vi "Terminal-DAQ-6133-Getter.vi"(8 "error in (no error)":errorcluster caption="错误输入（无错误）", 10 "读取次数":i32=160, 11 "write operation timeout (ms)":i32=5000 caption="写操作超时（5000毫秒）") -> (0 "error out":errorcluster caption="错误输出", 3 "6133":T1)   [LabVIEW 2014]
panel:
  in  "最大失败次数":i32=5
  out "失败次数":i32
  out "读取次数 2":i32
  in  "最大失败次数":i32=5
  in  "读取次数":i32=161
  out "error out":errorcluster caption="错误输出"
  in  "error in (no error)":errorcluster caption="错误输入（无错误）"
  in  "write operation timeout (ms)":i32=5000 caption="写操作超时（5000毫秒）"
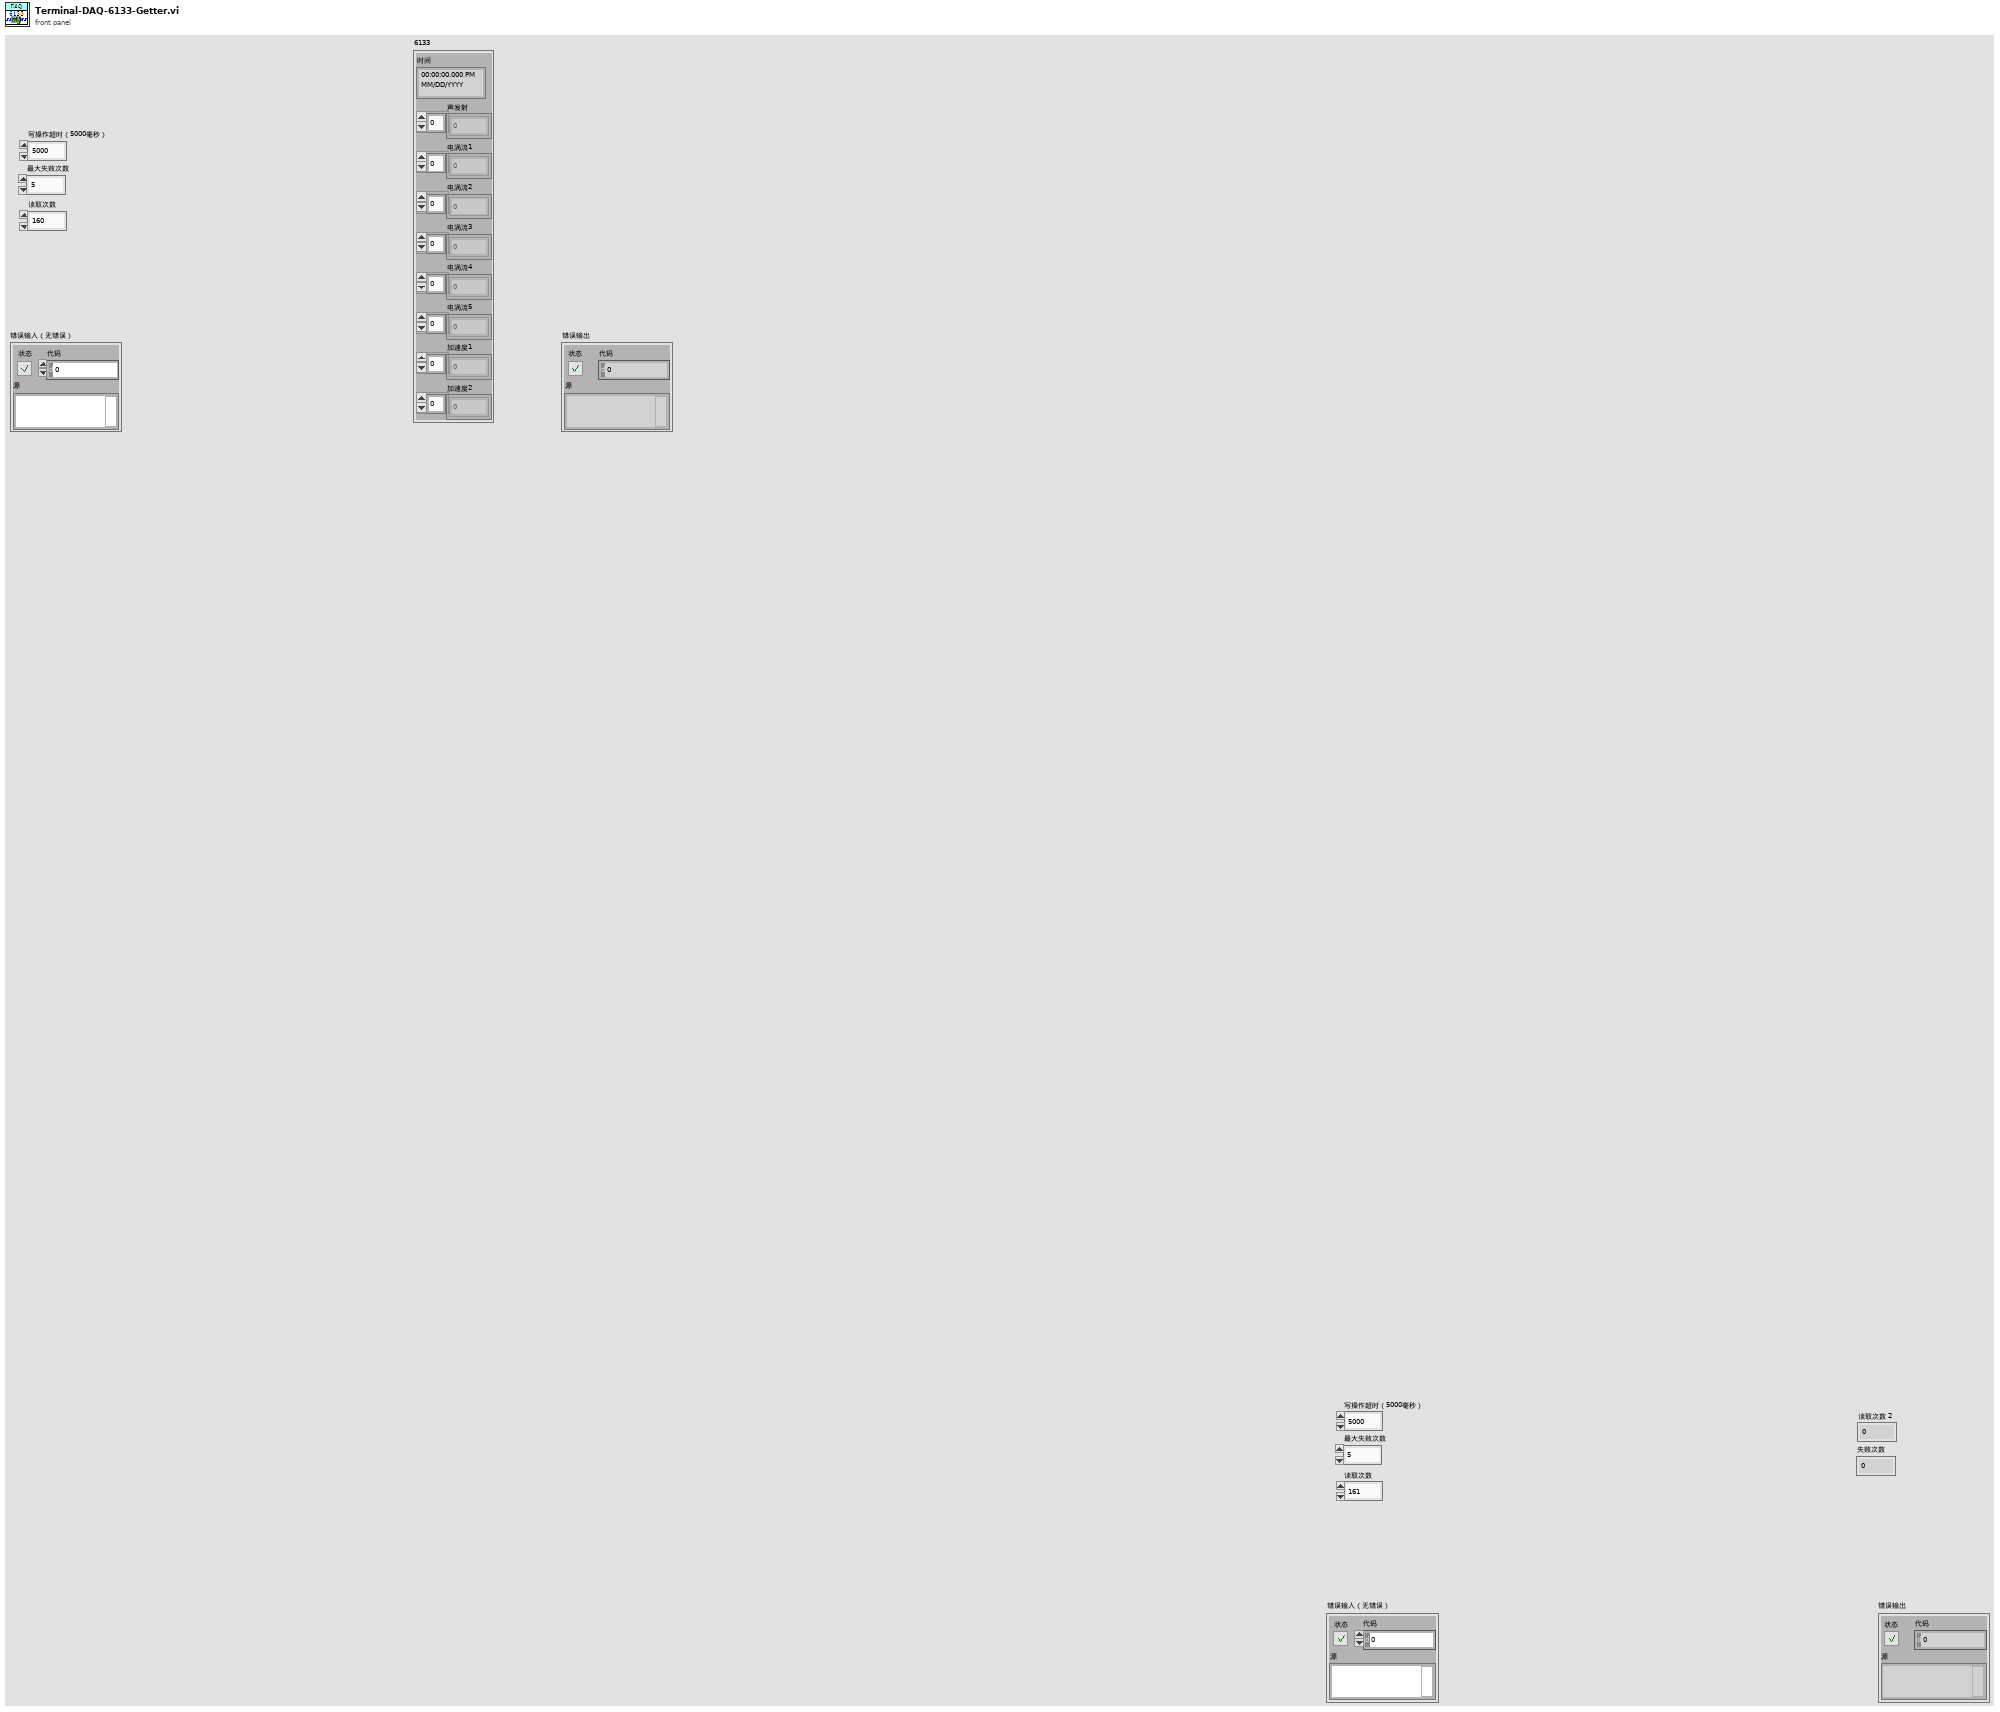
[diagram p1: front panel]
types:
  T1 = cluster{"时间":timestamp, "声发射":sgl[], "电涡流1":sgl[], "电涡流2":sgl[], "电涡流3":sgl[], "电涡流4":sgl[], "电涡流5":sgl[], "加速度1":sgl[], "加速度2":sgl[]}
  T2 = cluster{"设备名":string, "时间":timestamp, "数据":sgl[][], "通道长度":i32[], "次数":i32}
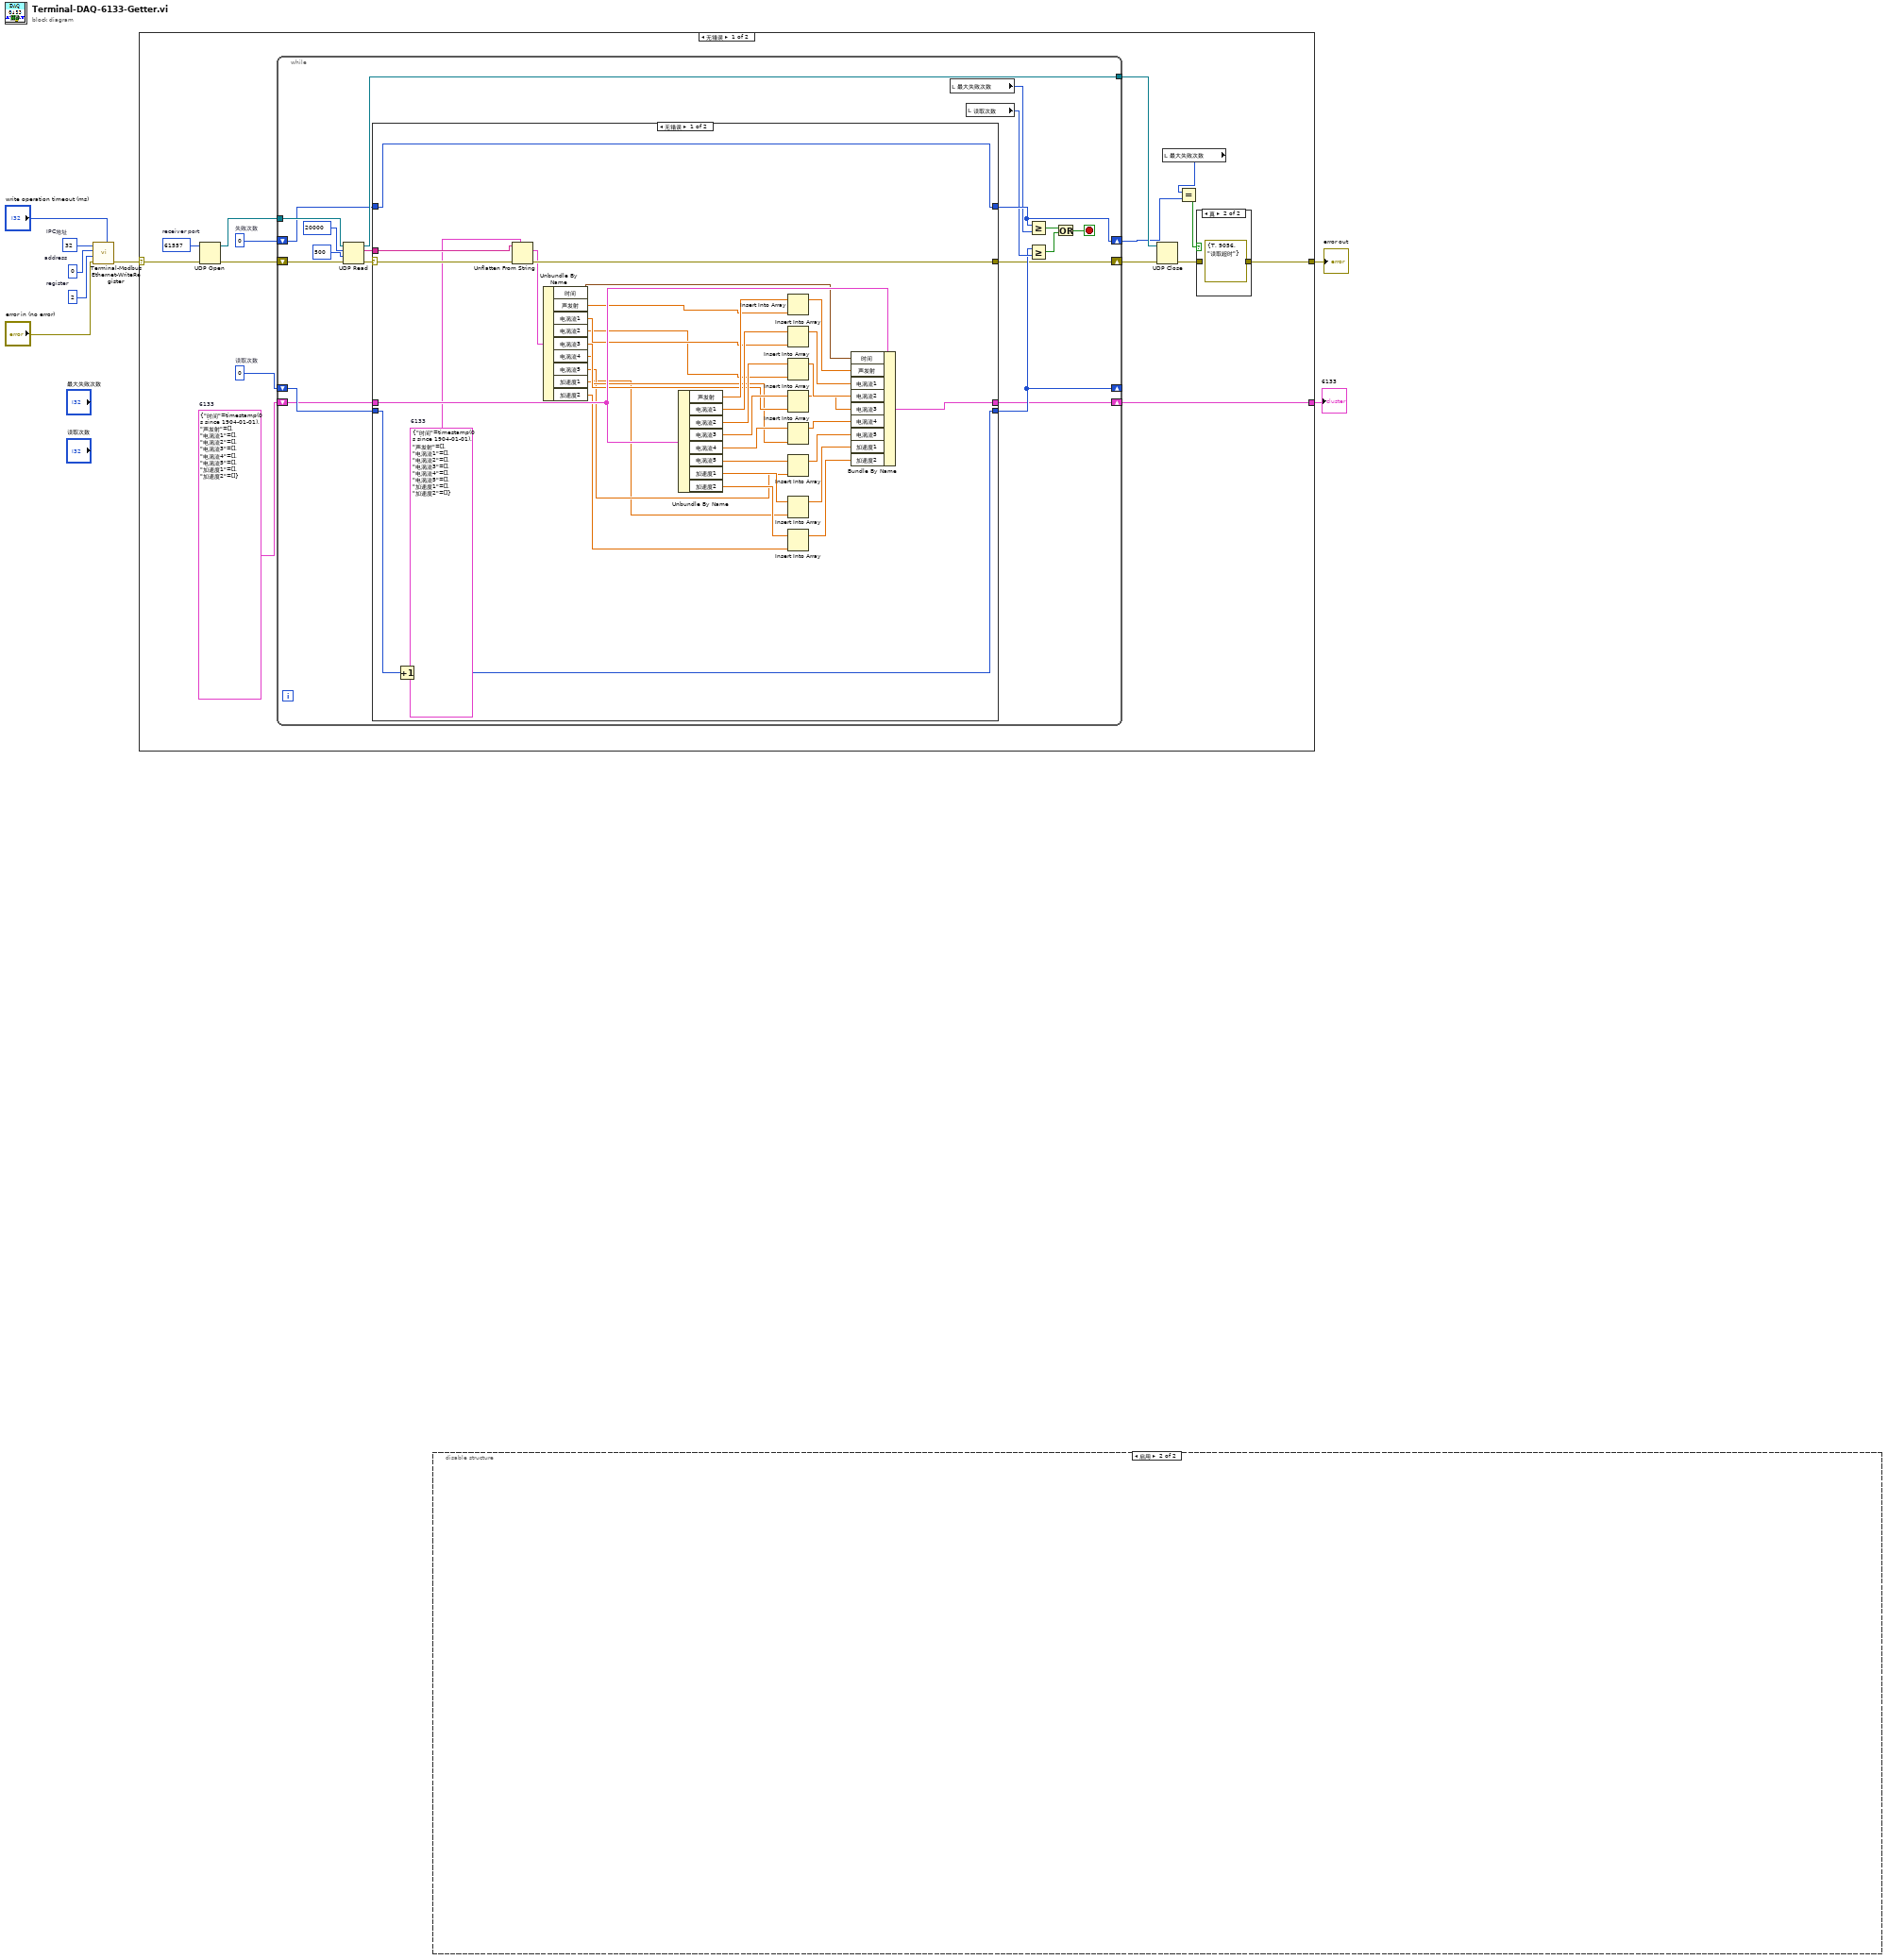
[diagram p0: block diagram]
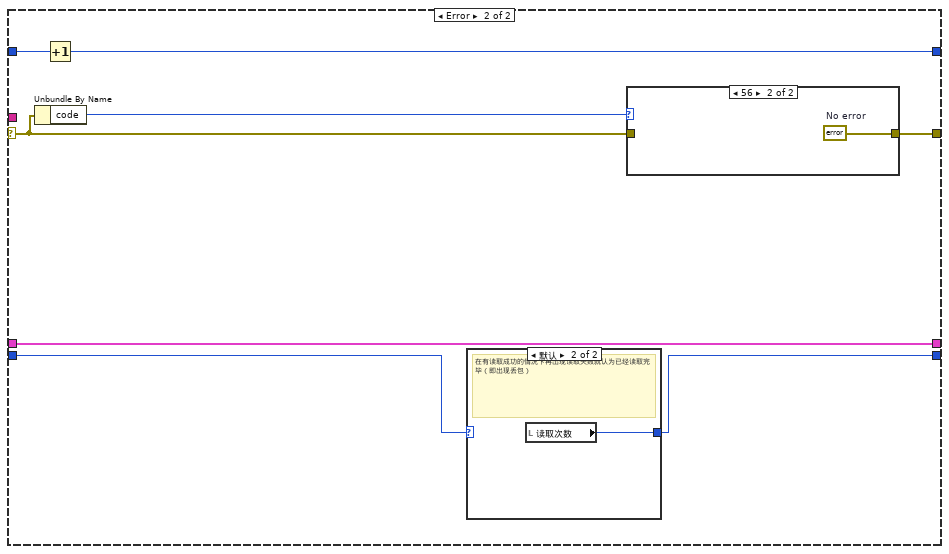
[diagram p3: hidden frame]
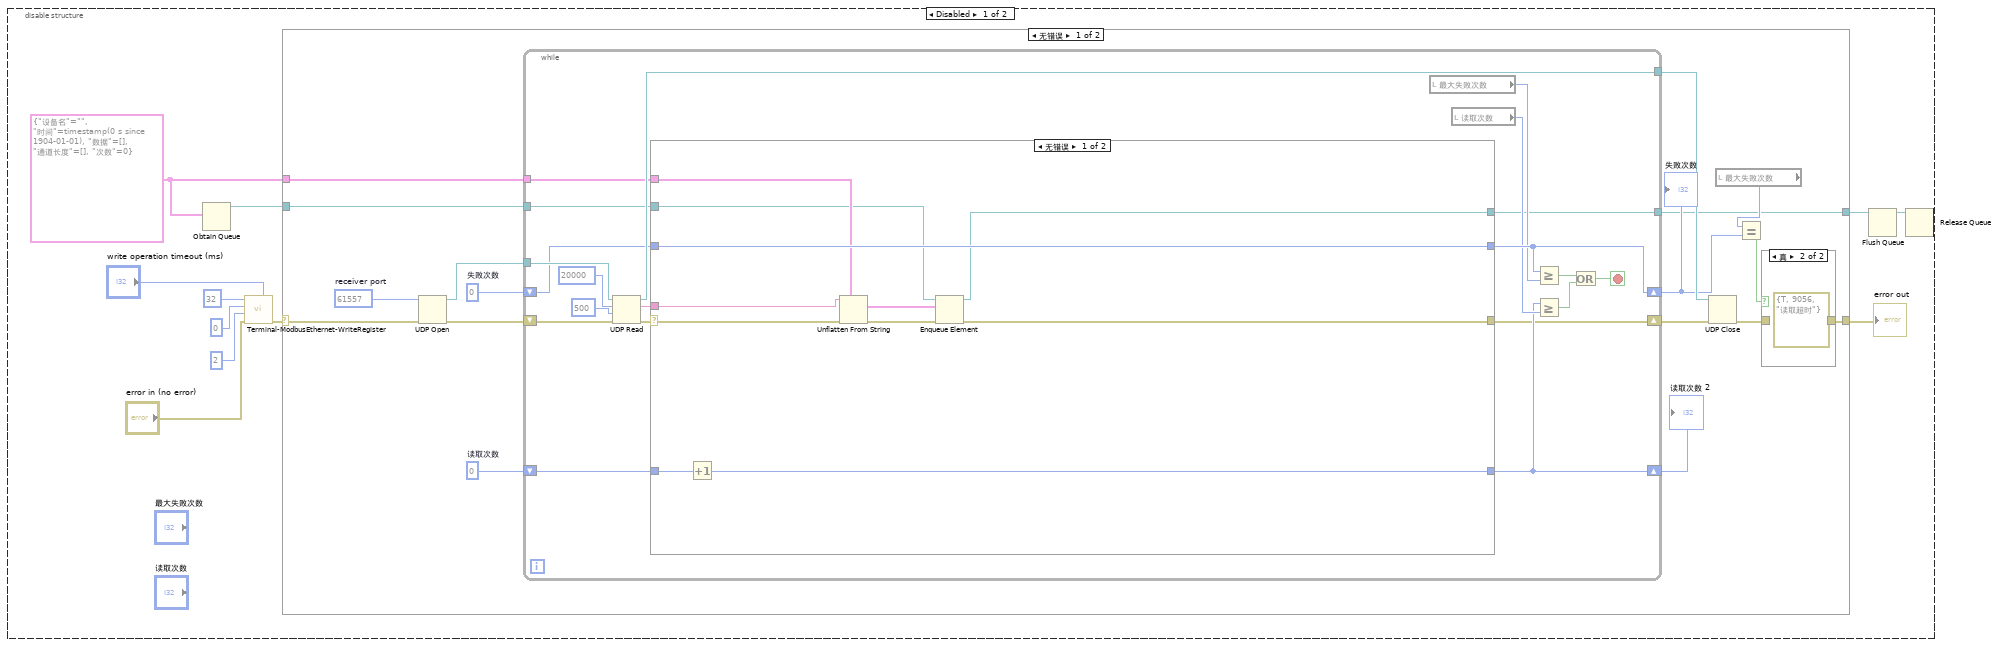
[diagram p7: hidden frame]
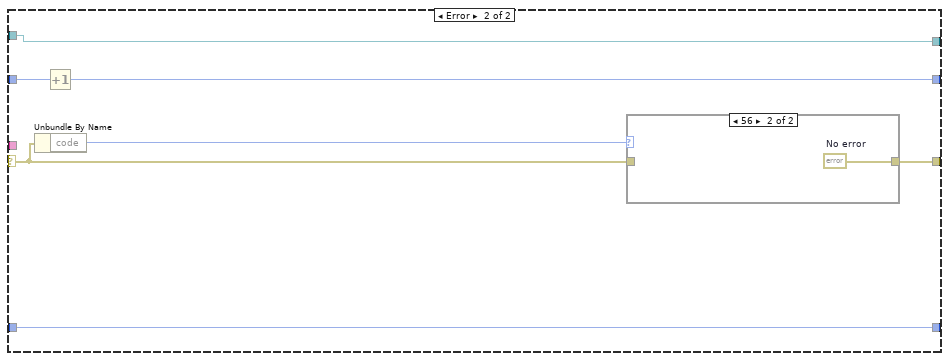
[diagram p9: hidden frame]
diagram:
  w4 = u16 2  # register
  w6 = u16 0  # address
  w5 = u8 32  # IPC地址
  n1 = call "Terminal-ModbusEthernet-WriteRegister.vi"("write operation timeout (ms)"="write operation timeout (ms)", "error in"="error in (no error)", "holding register value"=w4, "address"=w6, "unit ID"=w5) -> ("error out"=w3:errorcluster)  [unwired: 6 in]
  n2 = case shown="无错误" w3 {
    selector: w3 -> [w16 w92]
    tunnel: [w11 w92] -> w2
    tunnel: [w9 _] -> w1
    frame No Error {
      w10 = T1 {"时间"=timestamp(0 s since 1904-01-01), "声发射"=[], "电涡流1"=[], "电涡流2"=[], "电涡流3"=[], "电涡流4"=[], "电涡流5"=[], "加速度1"=[], "加速度2"=[]}  # 6133
      w17 = 0  # 读取次数
      w18 = 0  # 失败次数
      w23 = u16 61557  # receiver port
      n3 = UDP Open(8:w16, 11:w23) -> (port=w22:refnum<k16>, 0:w21:errorcluster)  [unwired: 3 in, 1 out]
      n4 = while {
        tunnel: w22 -> [w42]
        shift-right: [w28] -> w20
        shift-left: w21 -> [w41]
        tunnel: [w39] -> w19
        shift-right: [w36] -> w14
        shift-left: w18 -> [w37]
        shift-right: [w29] -> _
        shift-left: w17 -> [w35]
        shift-right: [w26] -> w9
        shift-left: w10 -> [w27]
        stop <- w31 stop-if-true
        n5 = UDP Read(connection ID=w42, max size (548)=20000 ("最大值(548)"), timeout ms (25000)=500, 8:w41) -> (data out=w38:string, error out=w40:errorcluster, 3:w39:refnum<k16>)  [unwired: 2 out]
        n6 = case shown="无错误" w40 {
          selector: w40 -> [w75 w85]
          tunnel: w38 -> [w79 _]
          tunnel: [w74 w86] -> w28
          tunnel: w37 -> [w76 w84]
          tunnel: [w76 w83] -> w36
          tunnel: w35 -> [w78 w81]
          tunnel: [w77 w80] -> w29
          tunnel: w27 -> [w73 w82]
          tunnel: [w71 w82] -> w26
          frame No Error {
            w53 = T1 {"时间"=timestamp(0 s since 1904-01-01), "声发射"=[], "电涡流1"=[], "电涡流2"=[], "电涡流3"=[], "电涡流4"=[], "电涡流5"=[], "加速度1"=[], "加速度2"=[]}  # 6133
            n7 = Increment(x=w78) -> (x+1=w77:i32)
            n8 = Unflatten From String(type=w53, binary string=w79, error in (no error)=w75) -> (value=w72:T1, error out=w74:errorcluster)  [unwired: 2 in, 1 out]
            n9 = Unbundle By Name(w72) -> ("时间"=w54:timestamp, "声发射"=w52:sgl[], "电涡流1"=w51:sgl[], "电涡流2"=w50:sgl[], "电涡流3"=w49:sgl[], "电涡流4"=w48:sgl[], "电涡流5"=w47:sgl[], "加速度1"=w46:sgl[], "加速度2"=w45:sgl[])
            n10 = Unbundle By Name(w73) -> ("声发射"=w70:sgl[], "电涡流1"=w69:sgl[], "电涡流2"=w68:sgl[], "电涡流3"=w67:sgl[], "电涡流4"=w66:sgl[], "电涡流5"=w65:sgl[], "加速度1"=w64:sgl[], "加速度2"=w63:sgl[])
            n11 = Insert Into Array(array=w70, new element=w52) -> (w55:sgl[])  [unwired: 1 in]
            n12 = Insert Into Array(array=w69, new element=w51) -> (w62:sgl[])  [unwired: 1 in]
            n13 = Insert Into Array(array=w68, new element=w50) -> (w61:sgl[])  [unwired: 1 in]
            n14 = Insert Into Array(array=w67, new element=w49) -> (w60:sgl[])  [unwired: 1 in]
            n15 = Insert Into Array(array=w66, new element=w48) -> (w59:sgl[])  [unwired: 1 in]
            n16 = Insert Into Array(array=w65, new element=w47) -> (w58:sgl[])  [unwired: 1 in]
            n17 = Insert Into Array(array=w64, new element=w46) -> (w57:sgl[])  [unwired: 1 in]
            n18 = Insert Into Array(array=w63, new element=w45) -> (w56:sgl[])  [unwired: 1 in]
            n19 = Bundle By Name(cluster=w73, "时间"=w54, "声发射"=w55, "电涡流1"=w62, "电涡流2"=w61, "电涡流3"=w60, "电涡流4"=w59, "电涡流5"=w58, "加速度1"=w57, "加速度2"=w56) -> (w71:T1)
          }
          frame Error {
            n20 = Unbundle By Name(w85) -> ("code"=w87:i32)
            n21 = Increment(x=w84) -> (x+1=w83:i32)
            n22 = case shown="默认" w81 {
              selector: w81 -> [w88 _]
              tunnel: [w88 w89] -> w80
              frame 0 {
              }
              frame Default {
                # "在有读取成功的情况下再出现读取失败就认为已经读取完毕（即出现丢包）"
                n23 = local read "读取次数"() -> (w89:i32)
              }
            }
            n24 = case shown="56" w87 {
              tunnel: w85 -> [w90 _]
              tunnel: [w90 w91] -> w86
              frame Default {
              }
              frame 56 {
                w91 = errorcluster {"status"=FALSE, "code"=0, "source"=""}  # No error
              }
            }
          }
        }
        n25 = local read "最大失败次数"() -> (w30:i32)
        n26 = local read "读取次数"() -> (w34:i32)
        n27 = Greater Or Equal?(x=w36, y=w30) -> (x >= y?=w33:bool)
        n28 = Greater Or Equal?(x=w29, y=w34) -> (x >= y?=w32:bool)
        n29 = Or(x=w33, y=w32) -> (x .or. y?=w31:bool)
      }
      n30 = UDP Close(connection ID=w19, 8:w20) -> (error out=w12:errorcluster)  [unwired: 1 out]
      n31 = local read "最大失败次数"() -> (w15:i32)
      n32 = Equal?(x=w15, y=w14) -> (x = y?=w13:bool)
      n33 = case shown="真" w13 {
        tunnel: w12 -> [w24 _]
        tunnel: [w24 errorcluster {"status"=TRUE, "code"=9056, "source"="读取超时"} ("错误常量")] -> w11
        frame False {
        }
        frame True {
        }
      }
    }
    frame Error {
    }
  }
  "error out" <- w2
  "6133" <- w1
  n34 = disable-structure shown="启用" {
    frame Disabled {
      w96 = T2 {"设备名"="", "时间"=timestamp(0 s since 1904-01-01), "数据"=[], "通道长度"=[], "次数"=0}
      n35 = Obtain Queue(element data type=w96) -> (queue out=w95:refnum<queue>)  [unwired: 4 in, 2 out]
      n36 = call "Terminal-ModbusEthernet-WriteRegister.vi"("write operation timeout (ms)"="write operation timeout (ms)", "error in"="error in (no error)", "holding register value"=u16 2 ("address"), "address"=u16 0, "unit ID"=u8 32) -> ("error out"=w98:errorcluster)  [unwired: 6 in]
      n37 = case shown="无错误" w98 {
        selector: w98 -> [w113 w164]
        tunnel: [w108 w164] -> w97
        tunnel: w96 -> [w107 _]
        tunnel: w95 -> [w106 w163]
        tunnel: [w105 w163] -> w94
        frame No Error {
          w114 = 0  # 读取次数
          w115 = 0  # 失败次数
          w120 = u16 61557  # receiver port
          n38 = UDP Open(8:w113, 11:w120) -> (port=w119:refnum<k16>, 0:w118:errorcluster)  [unwired: 3 in, 1 out]
          n39 = while {
            tunnel: w119 -> [w140]
            shift-right: [w126] -> w117
            shift-left: w118 -> [w139]
            tunnel: [w137] -> w116
            shift-right: [w134] -> w111
            shift-left: w115 -> [w135]
            shift-right: [w127] -> w104
            shift-left: w114 -> [w133]
            tunnel: w107 -> [w125]
            tunnel: w106 -> [w124]
            tunnel: [w123] -> w105
            stop <- w129 stop-if-true
            n40 = UDP Read(connection ID=w140, max size (548)=20000 ("最大值(548)"), timeout ms (25000)=500, 8:w139) -> (data out=w136:string, error out=w138:errorcluster, 3:w137:refnum<k16>)  [unwired: 2 out]
            n41 = case shown="无错误" w138 {
              selector: w138 -> [w150 w158]
              tunnel: w136 -> [w153 _]
              tunnel: [w144 w159] -> w126
              tunnel: w135 -> [w151 w157]
              tunnel: [w151 w156] -> w134
              tunnel: w133 -> [w149 w155]
              tunnel: [w152 w155] -> w127
              tunnel: w125 -> [w148 _]
              tunnel: w124 -> [w147 w154]
              tunnel: [w143 w154] -> w123
              frame No Error {
                n42 = Increment(x=w149) -> (x+1=w152:i32)
                n43 = Unflatten From String(type=w148, binary string=w153, error in (no error)=w150) -> (value=w146:T2, error out=w145:errorcluster)  [unwired: 2 in, 1 out]
                n44 = Enqueue Element(queue=w147, element=w146, error in (no error)=w145) -> (queue out=w143:refnum<queue>, error out=w144:errorcluster)  [unwired: 1 in, 1 out]
              }
              frame Error {
                n45 = Unbundle By Name(w158) -> ("code"=w160:i32)
                n46 = Increment(x=w157) -> (x+1=w156:i32)
                n47 = case shown="56" w160 {
                  tunnel: w158 -> [w161 _]
                  tunnel: [w161 w162] -> w159
                  frame Default {
                  }
                  frame 56 {
                    w162 = errorcluster {"status"=FALSE, "code"=0, "source"=""}  # No error
                  }
                }
              }
            }
            n48 = local read "最大失败次数"() -> (w128:i32)
            n49 = local read "读取次数"() -> (w132:i32)
            n50 = Greater Or Equal?(x=w134, y=w128) -> (x >= y?=w131:bool)
            n51 = Greater Or Equal?(x=w127, y=w132) -> (x >= y?=w130:bool)
            n52 = Or(x=w131, y=w130) -> (x .or. y?=w129:bool)
          }
          "读取次数 2" <- w104
          "失败次数" <- w111
          n53 = UDP Close(connection ID=w116, 8:w117) -> (error out=w109:errorcluster)  [unwired: 1 out]
          n54 = local read "最大失败次数"() -> (w112:i32)
          n55 = Equal?(x=w112, y=w111) -> (x = y?=w110:bool)
          n56 = case shown="真" w110 {
            tunnel: w109 -> [w121 _]
            tunnel: [w121 errorcluster {"status"=TRUE, "code"=9056, "source"="读取超时"} ("错误常量")] -> w108
            frame False {
            }
            frame True {
            }
          }
        }
        frame Error {
        }
      }
      "error out" <- w97
      n57 = Flush Queue(queue=w94) -> (queue out=w93:refnum<queue>)  [unwired: 1 in, 2 out]
      n58 = Release Queue(queue=w93) -> ()  [unwired: 2 in, 3 out]
    }
    frame Enabled {
    }
  }
